vi "set_H2.vi"(1 "Manifold H2 Flow":dbl, 3 "H2 Active":bool, 5 "Remote":bool) -> ()   [LabVIEW 2011]
uses:
  low_level_proc/globals.vi
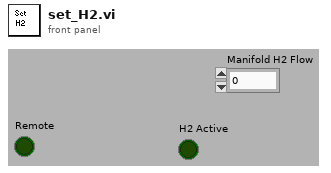
[diagram p1: front panel]
types:
  T1 = typedef "relaySpec.ctl" = cluster{"Card Index":u16, "Relay Index":u16}
  T2 = typedef "DA_Spec.ctl" = cluster{"Card Index":u16, "Channel Index":u16}
  T3 = typedef "AD_Spec.ctl" = u16
  T4 = cluster{"Relay Functions":cluster{"Remote":T1, "H2 active":T1, "N2 active":T1, "Output":T1}, "D/A Functions":cluster{"H2 flow":T2, "N2 flow":T2}, "Flow Ranges":cluster{"H2 flow (HMFC1)":u16, "N2 flow (NMFC1)":u16}, "A/D Functions":cluster{"H2/N2 flow":T3}}
  T5 = cluster{"Remote":T1, "H2 active":T1, "N2 active":T1, "Output":T1}
  T6 = cluster{"H2 flow (HMFC1)":u16, "N2 flow (NMFC1)":u16}
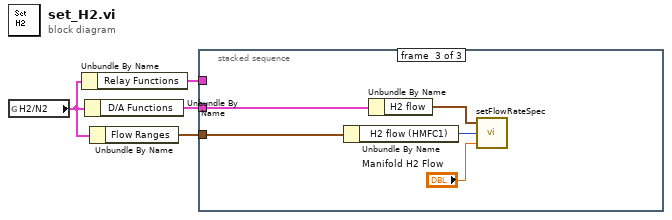
[diagram p0: block diagram]
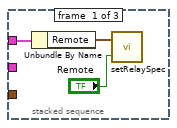
[diagram p2: hidden frame]
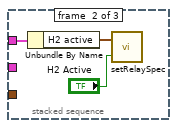
[diagram p3: hidden frame]
diagram:
  n1 = global read "globals.vi" "H2/N2"() -> (w2:T4)
  n2 = Unbundle By Name(w2) -> ("Relay Functions"=w4:T5)
  n3 = Unbundle By Name(w2) -> ("D/A Functions"=w3:cluster{"H2 flow":T2, "N2 flow":T2})
  n4 = Unbundle By Name(w2) -> ("Flow Ranges"=w1:T6)
  n5 = stacked-sequence {
    tunnel: w4 -> [w7 w9 _]
    tunnel: w3 -> [_ _ w12]
    tunnel: w1 -> [_ _ w14]
    frame #0 {
      n6 = Unbundle By Name(w7) -> ("Remote"=w6:T1)
      n7 = call "setRelaySpec.vi"("Relay Status"="Remote", "RelaySpec"=w6) -> ()  [unwired: 1 in]
    }
    frame #1 {
      n8 = Unbundle By Name(w9) -> ("H2 active"=w8:T1)
      n9 = call "setRelaySpec.vi"("Relay Status"="H2 Active", "RelaySpec"=w8) -> ()  [unwired: 1 in]
    }
    frame #2 {
      n10 = Unbundle By Name(w14) -> ("H2 flow (HMFC1)"=w13:u16)
      n11 = Unbundle By Name(w12) -> ("H2 flow"=w11:T2)
      n12 = call "setFlowRateSpec.vi"("Flow Rate (sccm)"="Manifold H2 Flow", "Flow range Index"=w13, "D/A Card"=w11) -> ()  [unwired: 2 in]
    }
  }
